vi "practica8-tanque.vi"() -> ()   [LabVIEW 2013]
panel:
  in  "stop":bool
  in  "String":string
  in  "limite":dbl
  in  "desabilitar":bool
  in  "Boolean":bool
  in  "posicion horizontal del tanque":dbl(slide) scale=0.0..400.0
  out "tanque":dbl(slide) scale=0.0..10.0
  in  "posicion vertical del tanque":dbl(slide) scale=0.0..300.0
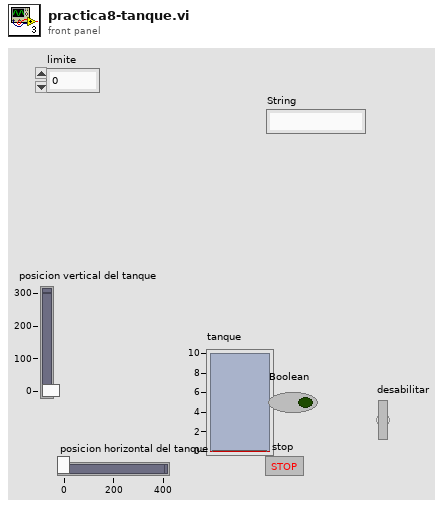
[diagram p1: front panel]
types:
  T1 = cluster{"posicion horizontal del tanque":dbl, "posicion vertical del tanque":dbl}
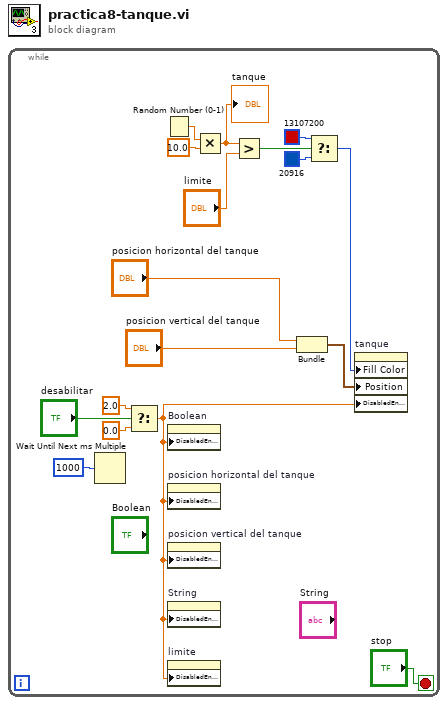
[diagram p0: block diagram]
diagram:
  n1 = while {
    stop <- "stop" stop-if-true
    n2 = Wait Until Next ms Multiple(millisecond multiple=u32 1000) -> ()  [unwired: 1 out]
    n3 = Select(t=2.0, s="desabilitar", f=0.0) -> (s? t:f=w2:dbl)
    n4 = Random Number (0-1)() -> (number: 0 to 1=w17:dbl)
    n5 = property on="Boolean" class="Bool (strict)"("DisabledEnum"=w2) -> ()  [unwired: 2 in, 2 out]
    n6 = property on="posicion horizontal del tanque" class="Slide (strict)"("DisabledEnum"=w2) -> ()  [unwired: 2 in, 2 out]
    n7 = property on="posicion vertical del tanque" class="Slide (strict)"("DisabledEnum"=w2) -> ()  [unwired: 2 in, 2 out]
    n8 = property on="String" class="Str"("DisabledEnum"=w2) -> ()  [unwired: 2 in, 2 out]
    n9 = property on="limite" class="DigNum (strict)"("DisabledEnum"=w2) -> ()  [unwired: 2 in, 2 out]
    n10 = Multiply(x=w17, y=10.0) -> (x*y=w14:dbl)
    "tanque" <- w14
    n11 = Greater?(x=w14, y="limite") -> (0:w13:bool)
    n12 = Bundle("posicion horizontal del tanque"="posicion horizontal del tanque", "posicion vertical del tanque"="posicion vertical del tanque") -> (w6:T1)  [unwired: 1 in]
    n13 = Select(t=u32 13107200, s=w13, f=u32 20916) -> (s? t:f=w7:u32)
    n14 = property on="tanque" class="Slide (strict)"("Fill Color"=w7, "Position"=w6, "DisabledEnum"=w2) -> ()  [unwired: 2 in, 2 out]
  }
